vi "Impedance fix.vi"() -> ()   [LabVIEW 2016]
uses:
  <vilib>/Utility/file.llb/Write To Spreadsheet File (DBL).vi
  <vilib>/Utility/file.llb/Read From Spreadsheet File (DBL).vi
panel:
  in  "Current":string="p"
  in  "Group":string="p"
  in  "SigaChannels":string[](array[string])
  in  "Save Button":bool
  in  "Chan #":i32=-1
  out "Current":cluster{"all rows":dbl[], dbl[]}[](graph)
  in  "Divide by current chan #":i32=-1
  in  "Fequency":dbl=300000.0 format="%#_6p"
  in  "stop":bool
  in  "V -> Impedance ratio":dbl=100.0
  in  "C (parallel)":dbl(slide)=1e-09 scale=0.0..5e-09 scale format="%#_6p"
  in  "L (series)":dbl(slide) scale=0.0..1e-12 scale format="%#_6p"
  in  "Phase":dbl(slide) scale=-180.0..180.0
  out "Data and Fix":cluster{"all rows":dbl[], dbl[]}[](graph)
  in  "File path (dialog if empty)":path
  # "Column_X=chan # *2 +1\nColumn_Y=Column_X+1"
  # "Fix:  R=(I/V-Z_C^-1)^-1-Z_L"
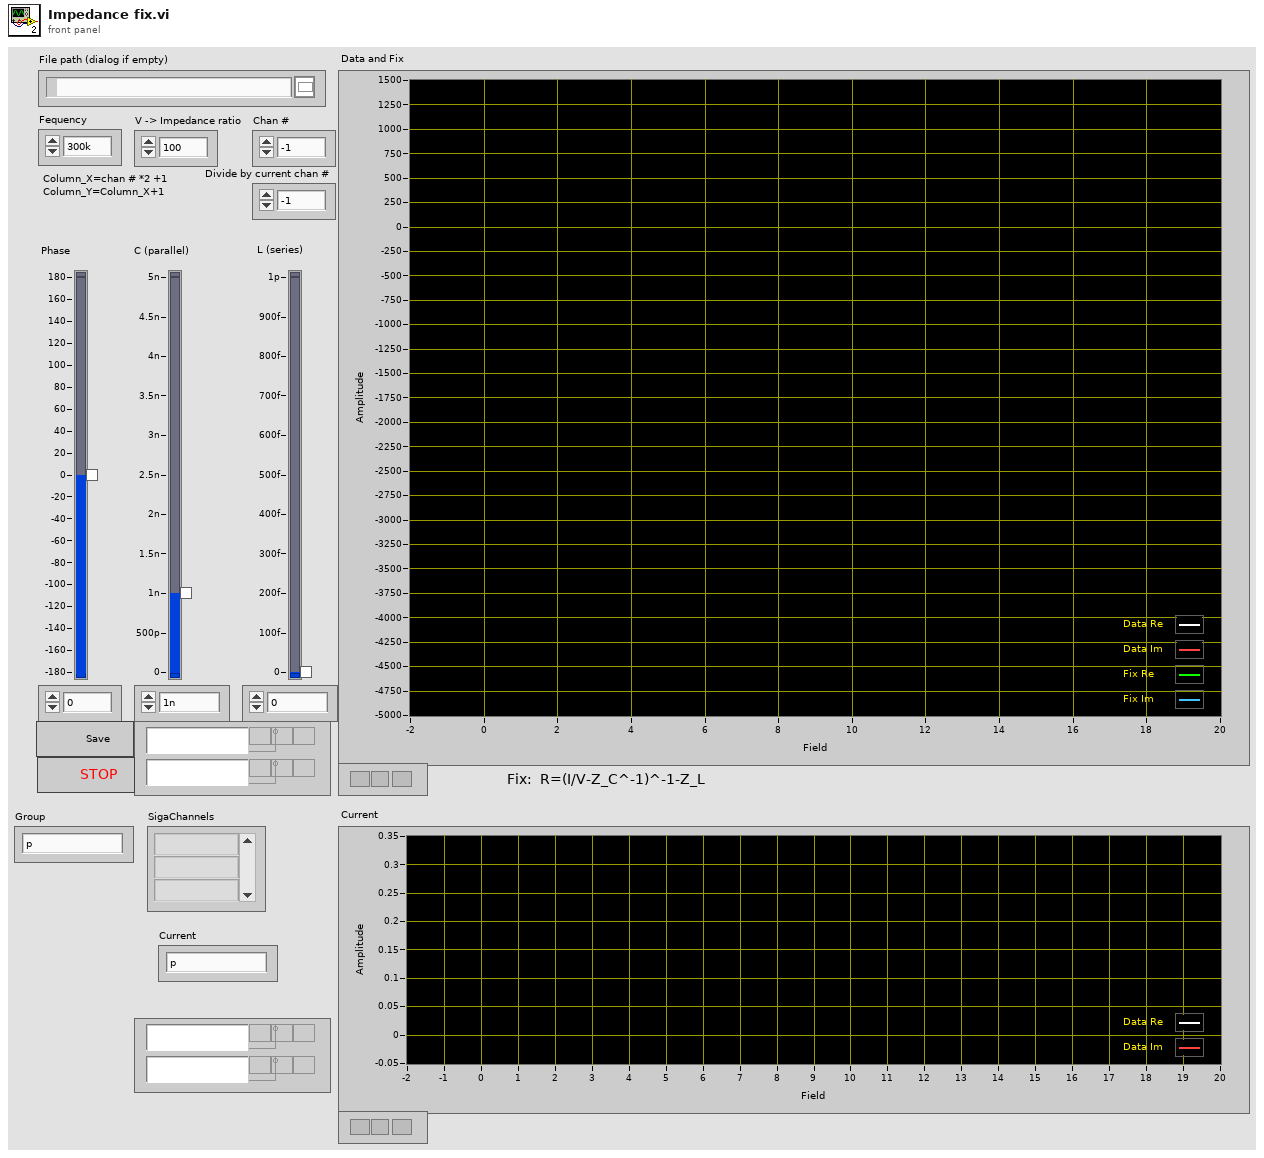
[diagram p1: front panel]
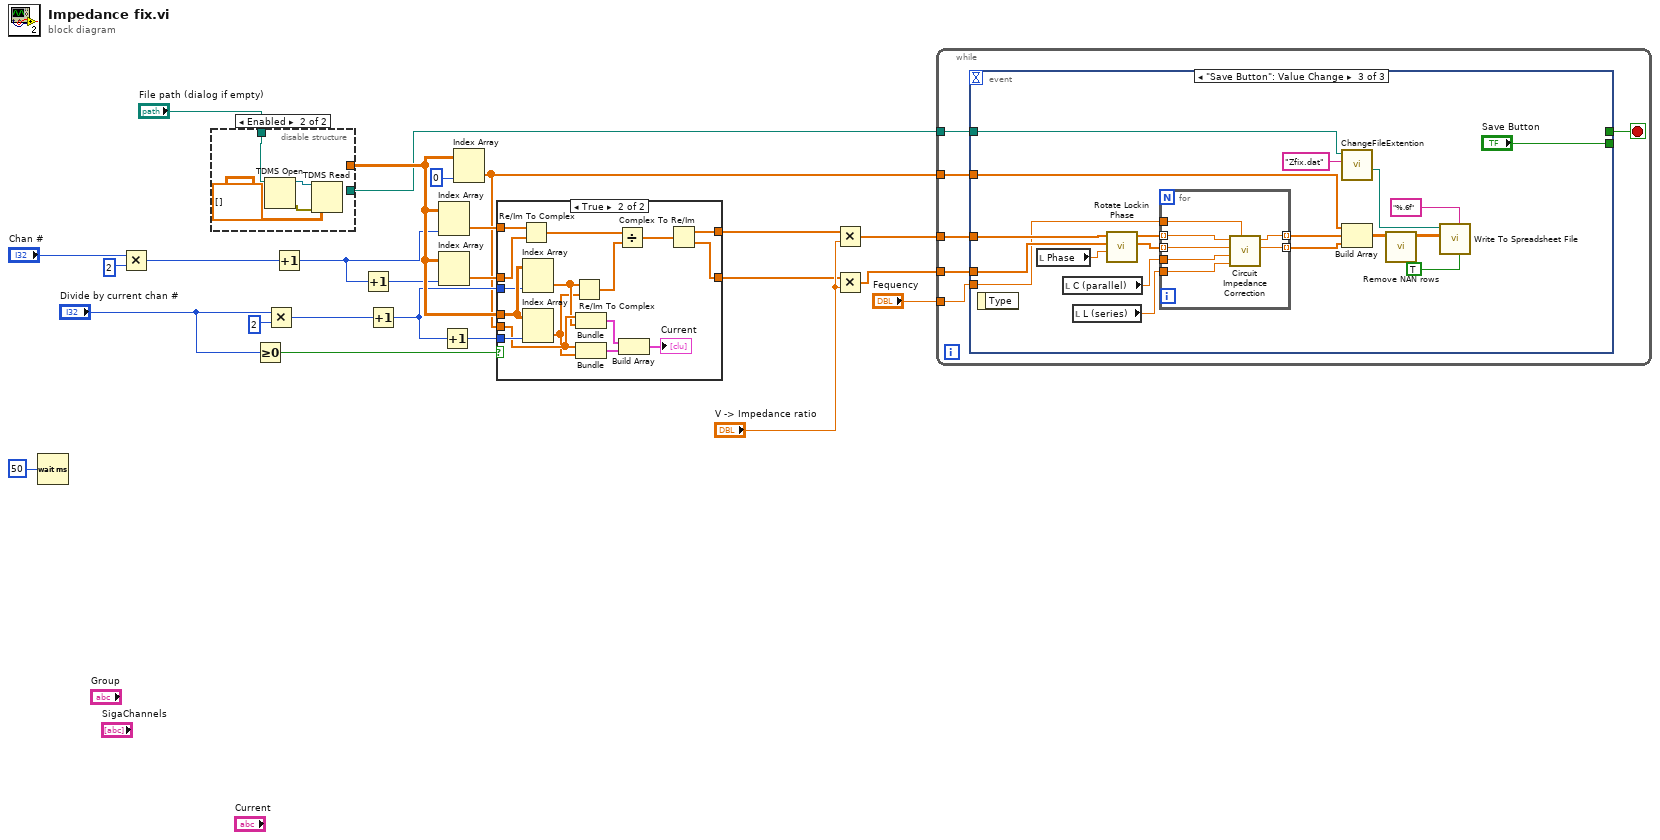
[diagram p0: block diagram]
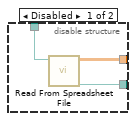
[diagram p2: hidden frame]
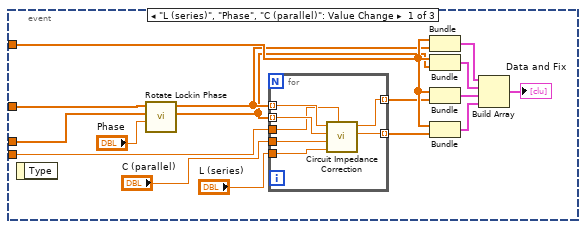
[diagram p4: hidden frame]
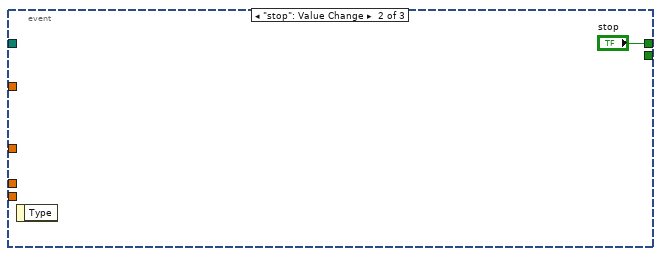
[diagram p5: hidden frame]
diagram:
  n1 = Wait (ms)(milliseconds to wait=u32 50) -> ()  [unwired: 1 out]
  n2 = Multiply(x="Chan #", y=2) -> (x*y=w7:i32)
  n3 = disable-structure shown="Enabled" {
    disable-tunnel: "File path (dialog if empty)" -> [w28 w32]
    disable-tunnel: [w27 _] -> w15
    disable-tunnel: [w26 _] -> w1
    frame Disabled {
      n4 = call-poly <vilib>:"Read From Spreadsheet File.vi"("file path (dialog if empty)"=w28) -> ("all rows"=w27:dbl[][], "new file path (Not A Path if cancelled)"=w26:path)  [unwired: 6 in, 3 out]
    }
    frame Enabled {
      n5 = TDMS Open(11:w32) -> (0:w30:errorcluster, 3:w31:refnum<k34>)  [unwired: 6 in]
      n6 = TDMS Read(0:w31, 11:w30, 12:dbl[][] [] ("all rows")) -> ()  [unwired: 5 in, 6 out]
    }
  }
  n7 = Greater Or Equal To 0?(x="Divide by current chan #") -> (x >= 0?=w9:bool)
  n8 = Multiply(x="Divide by current chan #", y=2) -> (x*y=w12:i32)
  n9 = Increment(x=w7) -> (x+1=w5:i32)
  n10 = Increment(x=w5) -> (x+1=w4:i32)
  n11 = Increment(x=w12) -> (x+1=w11:i32)
  n12 = Index Array(array=w15, index (col)=w5) -> (element=w19:dbl[])  [unwired: 1 in]
  n13 = Index Array(array=w15, index (col)=w4) -> (element=w17:dbl[])  [unwired: 1 in]
  n14 = Increment(x=w11) -> (x+1=w10:i32)
  n15 = Index Array(array=w15, index (col)=0 ("disabled index (col)")) -> (element=w8:dbl[])  [unwired: 1 in]
  n16 = case shown="True" w9 {
    tunnel: w19 -> [w34 w47]
    tunnel: [w34 w42] -> w18
    tunnel: w17 -> [w33 w46]
    tunnel: [w33 w41] -> w16
    tunnel: w15 -> [_ w50]
    tunnel: w11 -> [_ w49]
    tunnel: w10 -> [_ w48]
    tunnel: w8 -> [_ w38]
    frame False {
    }
    frame True {
      n17 = Re/Im To Complex(1:w46, 2:w47) -> (0:w45:cdb[])
      n18 = Index Array(array=w50, index (col)=w49) -> (element=w37:dbl[])  [unwired: 1 in]
      n19 = Index Array(array=w50, index (col)=w48) -> (element=w36:dbl[])  [unwired: 1 in]
      n20 = Re/Im To Complex(1:w36, 2:w37) -> (0:w44:cdb[])
      n21 = Bundle("all rows"=w38, "all rows"=w37) -> (w40:cluster{"all rows":dbl[], "all rows":dbl[]})  [unwired: 1 in]
      n22 = Bundle("all rows"=w38, "all rows"=w36) -> (w39:cluster{"all rows":dbl[], "all rows":dbl[]})  [unwired: 1 in]
      n23 = Divide(x=w45, y=w44) -> (x/y=w43:cdb[])
      n24 = Build Array(w40, w39) -> (→"Current":cluster{"all rows":dbl[], "all rows":dbl[]}[])
      n25 = Complex To Re/Im(x + iy=w43) -> (x=w42:dbl[], y=w41:dbl[])
    }
  }
  n26 = Multiply(x=w18, y="V -> Impedance ratio") -> (x*y=w23:dbl[])
  n27 = Multiply(x=w16, y="V -> Impedance ratio") -> (x*y=w22:dbl[])
  n28 = while {
    tunnel: w23 -> [w53]
    tunnel: w22 -> [w52]
    tunnel: w8 -> [w56]
    tunnel: "Fequency" -> [w54]
    tunnel: w1 -> [w51]
    stop <- w55 stop-if-true
    n29 = event shown="[2] \"Save Button\": Value Change" {
      selector: _ -> [_ _ _]
      dyn-events: _ -> [_ _ _]
      timeout: _ -> [_ _ _]
      tunnel: w56 -> [w72 _ w85]
      tunnel: [_ "stop" _] -> w55
      tunnel: w54 -> [w68 _ w91]
      tunnel: w53 -> [w60 _ w95]
      tunnel: w52 -> [w58 _ w94]
      tunnel: [_ _ "Save Button"] -> _
      tunnel: w51 -> [_ _ w89]
      event "L (series)", "Phase", "C (parallel)": Value Change {
        n30 = event-data() -> ()  [unwired: 1 in, 1 out]
        n31 = call "Rotate Lockin Phase.vi"("Phase"="Phase", "Array Y in"=w58, "Array X in"=w60) -> ("Array Y out"=w57:dbl[], "Array X out"=w59:dbl[])  [unwired: 7 out]
        n32 = for {
          tunnel: w59 -> [w79] mode=indexing
          tunnel: w57 -> [w78] mode=indexing
          tunnel: "C (parallel)" -> [w77]
          tunnel: w68 -> [w76]
          tunnel: "L (series)" -> [w75]
          tunnel: [w74] -> w66 mode=indexing
          tunnel: [w73] -> w65 mode=indexing
          n33 = call "Circuit Impedance Correction.vi"("Fequency"=w76, "Series inductance"=w75, "Parallel capacitance"=w77, "Measured Resistance Y"=w78, "Measured Resistance X"=w79) -> ("Corrected resistance Y"=w73:dbl, "Corrected resistance X"=w74:dbl)  [unwired: 4 in, 1 out]
        }
        n34 = Bundle("all rows"=w72, "Array X out"=w59) -> (w71:cluster{"all rows":dbl[], "Array X out":dbl[]})  [unwired: 1 in]
        n35 = Bundle("all rows"=w72, "Array Y out"=w57) -> (w70:cluster{"all rows":dbl[], "Array Y out":dbl[]})  [unwired: 1 in]
        n36 = Bundle("all rows"=w72, w66) -> (w64:cluster{"all rows":dbl[], dbl[]})  [unwired: 1 in]
        n37 = Bundle("all rows"=w72, w65) -> (w63:cluster{"all rows":dbl[], dbl[]})  [unwired: 1 in]
        n38 = Build Array(w71, w70, w64, w63) -> (→"Data and Fix":cluster{"all rows":dbl[], "Array Y out":dbl[]}[])
      }
      event "stop": Value Change {
        n39 = event-data() -> ()  [unwired: 1 in, 1 out]
      }
      event "Save Button": Value Change {
        n40 = event-data() -> ()  [unwired: 1 in, 1 out]
        n41 = local read "Phase"() -> (w96:dbl)
        n42 = local read "C (parallel)"() -> (w92:dbl)
        n43 = local read "L (series)"() -> (w93:dbl)
        n44 = call "Rotate Lockin Phase.vi"("Phase"=w96, "Array Y in"=w94, "Array X in"=w95) -> ("Array Y out"=w97:dbl[], "Array X out"=w98:dbl[])  [unwired: 7 out]
        n45 = for {
          tunnel: w98 -> [w106] mode=indexing
          tunnel: w97 -> [w105] mode=indexing
          tunnel: w92 -> [w104]
          tunnel: w91 -> [w103]
          tunnel: w93 -> [w102]
          tunnel: [w101] -> w84 mode=indexing
          tunnel: [w100] -> w83 mode=indexing
          n46 = call "Circuit Impedance Correction.vi"("Fequency"=w103, "Series inductance"=w102, "Parallel capacitance"=w104, "Measured Resistance Y"=w105, "Measured Resistance X"=w106) -> ("Corrected resistance Y"=w100:dbl, "Corrected resistance X"=w101:dbl)  [unwired: 4 in, 1 out]
        }
        n47 = call "ChangeFileExtention.vi"("New extension"="Zfix.dat" ("New Extention"), "File Path"=w89) -> ("Path with new extension"=w88:path)  [unwired: 2 in, 7 out]
        n48 = Build Array(w85, w84, w83) -> (w82:dbl[][])
        n49 = call "Remove NAN rows.vi"("Array - Numeric"=w82) -> ("Array out"=w81:dbl[][])  [unwired: 10 in]
        n50 = call-poly <vilib>:"Write To Spreadsheet File.vi"("transpose? (no:F)"=TRUE, "format (%.3f)"="%.6f", "2D data"=w81, "file path (dialog if empty)"=w88) -> ()  [unwired: 4 in, 1 out]
      }
    }
  }
